vi "Post.vi"(7 "Datum":refnum<class "Datum.lvclass">, 8 "Error In":errorcluster, 10 "Writer In":refnum<class "Writer.lvclass">, 11 "Render In":refnum<class "Process.lvclass">) -> (0 "Error Out":errorcluster, 2 "Writer Out":refnum<class "Writer.lvclass">, 3 "Render Out":refnum<class "Process.lvclass">)   [LabVIEW 2018, in "Toolkit.lvlib" / "Hooks.lvlib" / "Render.lvlib" / "Process.lvclass"]
uses:
  Process.lvclass
  Data/Datum/Datum.lvclass
  Low-Level/Writers/Writer/Writer.lvclass
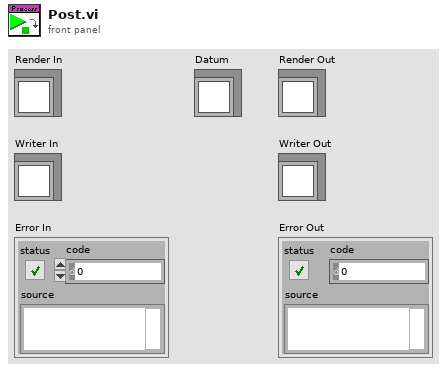
[diagram p1: front panel]
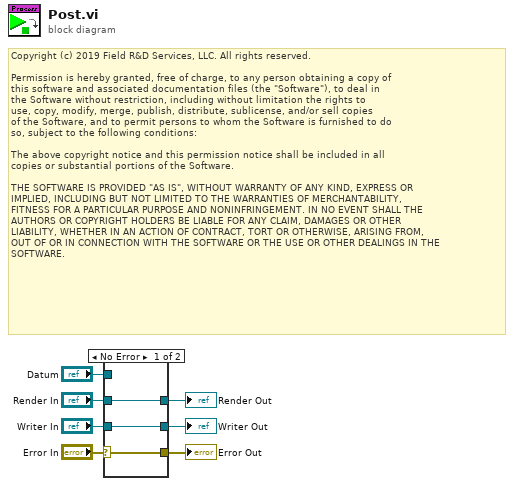
[diagram p0: block diagram]
diagram:
  # "Copyright (c) 2019 Field R&D Services, LLC. All rights reserved.\n\nPermission is hereby granted, free of charge, to any person obtaining a copy of\nthis software and associated documentation files (the \"Software\"), to deal in\nthe Software without restriction, including without limitation the rights to\nuse, copy, modify, merge, publish, distribute, sublicense, and/or sell copies\nof the Software, and to permit persons to whom the Software is furnished to do\nso, subject to the following conditions:\n\nThe above copyright notice and this permission notice shall be included in all\ncopies or substantial portions of the Software.\n\nTHE SOFTWARE IS PROVIDED \"AS IS\", WITHOUT WARRANTY OF ANY KIND, EXPRESS OR\nIMPLIED, INCLUDING BUT NOT LIMITED TO THE WARRANTIES OF MERCHANTABILITY,\nFITNESS FOR A PARTICULAR PURPOSE AND NONINFRINGEMENT. IN NO EVENT SHALL THE\nAUTHORS OR COPYRIGHT HOLDERS BE LIABLE FOR ANY CLAIM, DAMAGES OR OTHER\nLIABILITY, WHETHER IN AN ACTION OF CONTRACT, TORT OR OTHERWISE, ARISING FROM,\nOUT OF OR IN CONNECTION WITH THE SOFTWARE OR THE USE OR OTHER DEALINGS IN THE\nSOFTWARE."
  n1 = case shown="No Error" "Error In" {
    selector: "Error In" -> [w10 w12]
    tunnel: "Render In" -> [w9 w13]
    tunnel: [w9 w13] -> w6
    tunnel: [w10 w12] -> w4
    tunnel: "Writer In" -> [w8 w11]
    tunnel: [w8 w11] -> w1
    tunnel: "Datum" -> [_ _]
    frame No Error {
    }
    frame Error {
    }
  }
  "Render Out" <- w6
  "Error Out" <- w4
  "Writer Out" <- w1
